vi "PIV_VectorPlot.vi"(4 "xy scale":dbl=100.0 format="%#_13g", 6 "Offset":cluster{i32, i32}={10, 300}, 8 "color(black)":u32(colorbox), 9 "vector scale":dbl=0.05 format="%#_13g", 10 "picture":picture, 11 "velocities":T1) -> (3 "vectors":picture)   [LabVIEW 2025]
uses:
  PIV_velocities.ctl
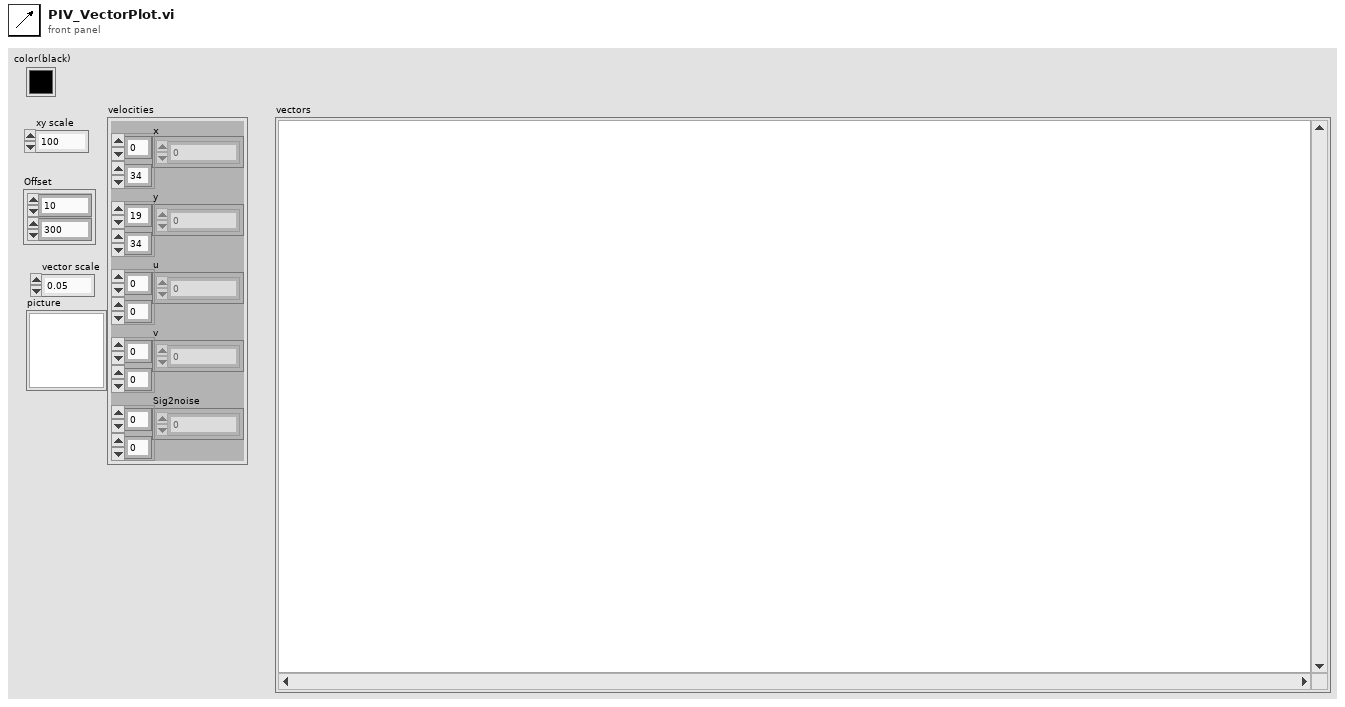
[diagram p1: front panel]
types:
  T1 = typedef "PIV_velocities.ctl" = cluster{"x":dbl[][], "y":dbl[][], "u":dbl[][], "v":dbl[][], "Sig2noise":dbl[][]}
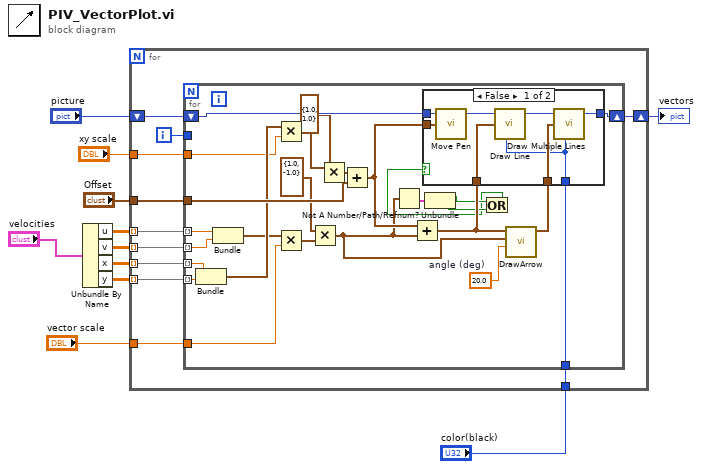
[diagram p0: block diagram]
diagram:
  n1 = Unbundle By Name("velocities") -> ("u"=w5:dbl[][], "v"=w6:dbl[][], "x"=w3:dbl[][], "y"=w2:dbl[][])
  n2 = for {
    tunnel: w5 -> [w22] mode=indexing
    tunnel: w6 -> [w21] mode=indexing
    shift-right: [w19] -> w8
    shift-left: "picture" -> [w20]
    tunnel: "Offset" -> [w17]
    tunnel: "vector scale" -> [w16]
    tunnel: "xy scale" -> [w15]
    tunnel: w3 -> [w14] mode=indexing
    tunnel: w2 -> [w13] mode=indexing
    tunnel: "color(black)" -> [w12]
    i -> [w18]
    n3 = for {
      tunnel: w22 -> [w47] mode=indexing
      tunnel: w21 -> [w46] mode=indexing
      shift-right: [w37] -> w19
      shift-left: w20 -> [w48]
      tunnel: w18 -> [_]
      tunnel: w17 -> [w45]
      tunnel: w16 -> [w43]
      tunnel: w15 -> [w42]
      tunnel: w14 -> [w36] mode=indexing
      tunnel: w13 -> [w35] mode=indexing
      tunnel: w12 -> [w23]
      w34 = 20.0  # angle (deg)
      n4 = Bundle(w36, w35) -> (w44:cluster{dbl, dbl})  [unwired: 1 in]
      n5 = Bundle(w47, w46) -> (w32:cluster{dbl, dbl})  [unwired: 1 in]
      n6 = Multiply(x=w44, y=w42) -> (x*y=w40:cluster{dbl, dbl})
      n7 = Multiply(x=w32, y=w43) -> (x*y=w30:cluster{dbl, dbl})
      n8 = Multiply(x=cluster{dbl, dbl} {1.0, -1.0} ("y"), y=w30) -> (x*y=w29:cluster{dbl, dbl})
      n9 = Multiply(x=w40, y=cluster{dbl, dbl} {1.0, 1.0}) -> (x*y=w39:cluster{dbl, dbl})
      n10 = Add(x=w39, y=w45) -> (x+y=w41:cluster{dbl, dbl})
      n11 = Not A Number/Path/Refnum?(number/path/refnum=w29) -> (NaN/Path/Refnum?=w28:cluster{bool, bool})
      n12 = Add(x=w41, y=w29) -> (x+y=w31:cluster{dbl, dbl})
      n13 = Unbundle(w28) -> (w27:bool, w26:bool)
      n14 = Or(x=w27, y=w26) -> (x .or. y?=w25:bool)
      n15 = call "DrawArrow.vi"("angle (deg)"=w34, "velocity"=w29, "end of line"=w31) -> ("arrow"=w33:cluster{dbl, dbl}[])  [unwired: 8 in]
      n16 = case shown="False" w25 {
        tunnel: w48 -> [w56 w57]
        tunnel: w41 -> [w54 _]
        tunnel: [w52 w57] -> w37
        tunnel: w33 -> [w51 _]
        tunnel: w31 -> [w50 _]
        tunnel: w23 -> [w49 _]
        frame False {
          n17 = call <vilib>:"Move Pen.vi"("new position"=w54, "picture"=w56) -> ("new picture"=w55:picture)  [unwired: 3 in]
          n18 = call <vilib>:"Draw Line.vi"("picture"=w55, "end point"=w50, "color(black)"=w49) -> ("new picture"=w53:picture)  [unwired: 6 in]
          n19 = call <vilib>:"Draw Multiple Lines.vi"("picture"=w53, "line endpoints"=w51, "color(black)"=w49) -> ("new picture"=w52:picture)  [unwired: 6 in]
        }
        frame True {
        }
      }
    }
  }
  "vectors" <- w8
